vi "Top - 1.vi"(0 "OPC UA client refnum out":T1, 9 "stop":bool, 11 "error IO":errorcluster) -> (3 "Az":T2, 4 "Alt":T3, 6 "HSB":T4, 8 "Fork Panel":T5, 10 "UPS":T7, 15 "Alarm Warning":T8)   [LabVIEW 2019]
uses:
  subVIs/Alarm-Ctrl.ctl
  subVIs/UPS-Ctrl.ctl
  <vilib>/OPCUA/controls/NodeId.ctl
  subVIs/Fork Panel-Ctrl.ctl
  subVIs/HSB-Ctrl.ctl
  subVIs/Alt-Ctrl.ctl
  subVIs/Az-Ctrl.ctl
  <vilib>/OPCUA/controls/OPC UA Client Refnum.ctl
  <vilib>/OPCUA/controls/Write Variant Request.ctl
  <vilib>/OPCUA/controls/Write Status.ctl
  <vilib>/OPCUA/client/Multiple Write Variant.vi
  <vilib>/OPCUA/NI OPC UA Client.lvlib
panel:
  in  "Device.Node.Set Point":i32=1000
  out "node RU":T6[](array[typedef])
  out "node RU 2":T6[](array[typedef])
  out "node RU 3":string[](array[string])
  # "Alarm Warning"
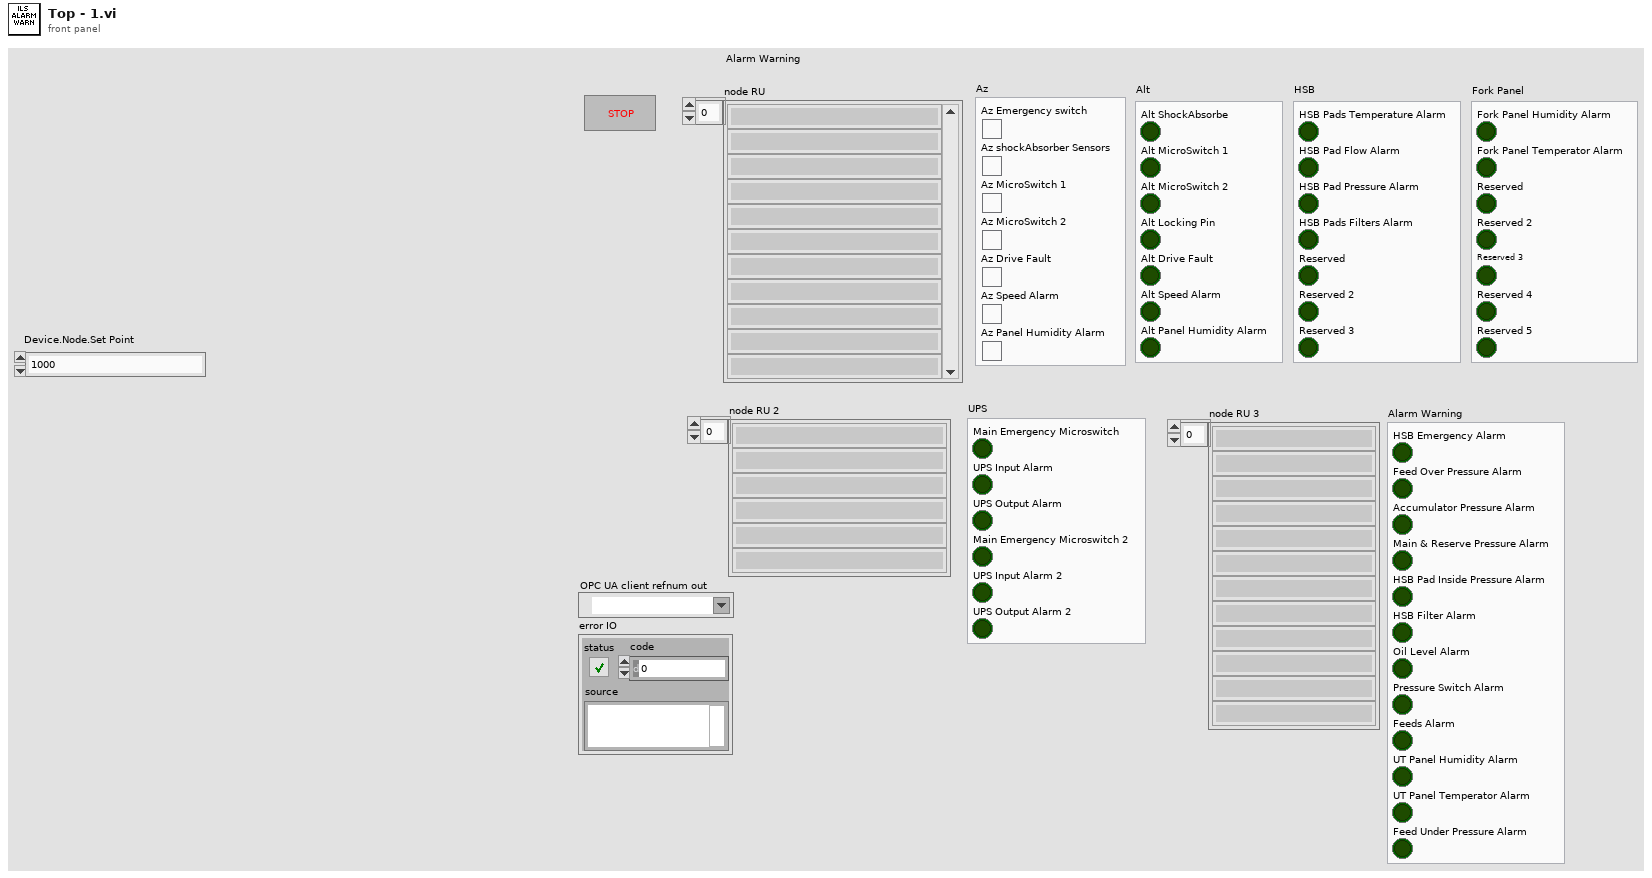
[diagram p1: front panel]
types:
  T1 = typedef "OPC UA Client Refnum.ctl" = refnum<k21>
  T2 = typedef "Az-Ctrl.ctl" = cluster{"Az Emergency switch":bool, "Az shockAbsorber Sensors":bool, "Az MicroSwitch 1":bool, "Az MicroSwitch 2":bool, "Az Drive Fault":bool, "Az Speed Alarm":bool, "Az Panel Humidity Alarm":bool}
  T3 = typedef "Alt-Ctrl.ctl" = cluster{"Alt ShockAbsorbe":bool, "Alt MicroSwitch 1":bool, "Alt MicroSwitch 2":bool, "Alt Locking Pin":bool, "Alt Drive Fault":bool, "Alt Speed Alarm":bool, "Alt Panel Humidity Alarm":bool}
  T4 = typedef "HSB-Ctrl.ctl" = cluster{"HSB Pads Temperature Alarm":bool, "HSB Pad Flow Alarm":bool, "HSB Pad Pressure Alarm":bool, "HSB Pads Filters Alarm":bool, "Reserved":bool, "Reserved 2":bool, "Reserved 3":bool}
  T5 = typedef "Fork Panel-Ctrl.ctl" = cluster{"Fork Panel Humidity Alarm":bool, "Fork Panel Temperator Alarm":bool, "Reserved":bool, "Reserved 2":bool, "Reserved 3":bool, "Reserved 4":bool, "Reserved 5":bool}
  T6 = typedef "NodeId.ctl" = string
  T7 = typedef "UPS-Ctrl.ctl" = cluster{"Main Emergency Microswitch":bool, "UPS Input Alarm":bool, "UPS Output Alarm":bool, "Main Emergency Microswitch 2":bool, "UPS Input Alarm 2":bool, "UPS Output Alarm 2":bool}
  T8 = typedef "Alarm-Ctrl.ctl" = cluster{"HSB Emergency Alarm":bool, "Feed Over Pressure Alarm":bool, "Accumulator Pressure Alarm":bool, "Main & Reserve Pressure Alarm":bool, "HSB Pad Inside Pressure Alarm":bool, "HSB Filter Alarm":bool, "Oil Level Alarm":bool, "Pressure Switch Alarm":bool, "Feeds Alarm":bool, "UT Panel Humidity Alarm":bool, "UT Panel Temperator Alarm":bool, "Feed Under Pressure Alarm":bool}
  T9 = typedef "Write Variant Request.ctl" = cluster{"node ID":T6, "value":variant, "timestamp (current time)":timestamp, "node status":T10}
  T10 = typedef "Write Status.ctl" = u32
  T11 = typedef "Subscription ID.ctl" = u32
  T12 = typedef "Subscription Data Change.ctl" = cluster{"node ID":T6, " value":variant, "timestamp":timestamp, "data type":T13, "status code":T14}
  T13 = typedef "Data Type.ctl" = u16
  T14 = typedef "OPC UA StatusCode.ctl" = u32
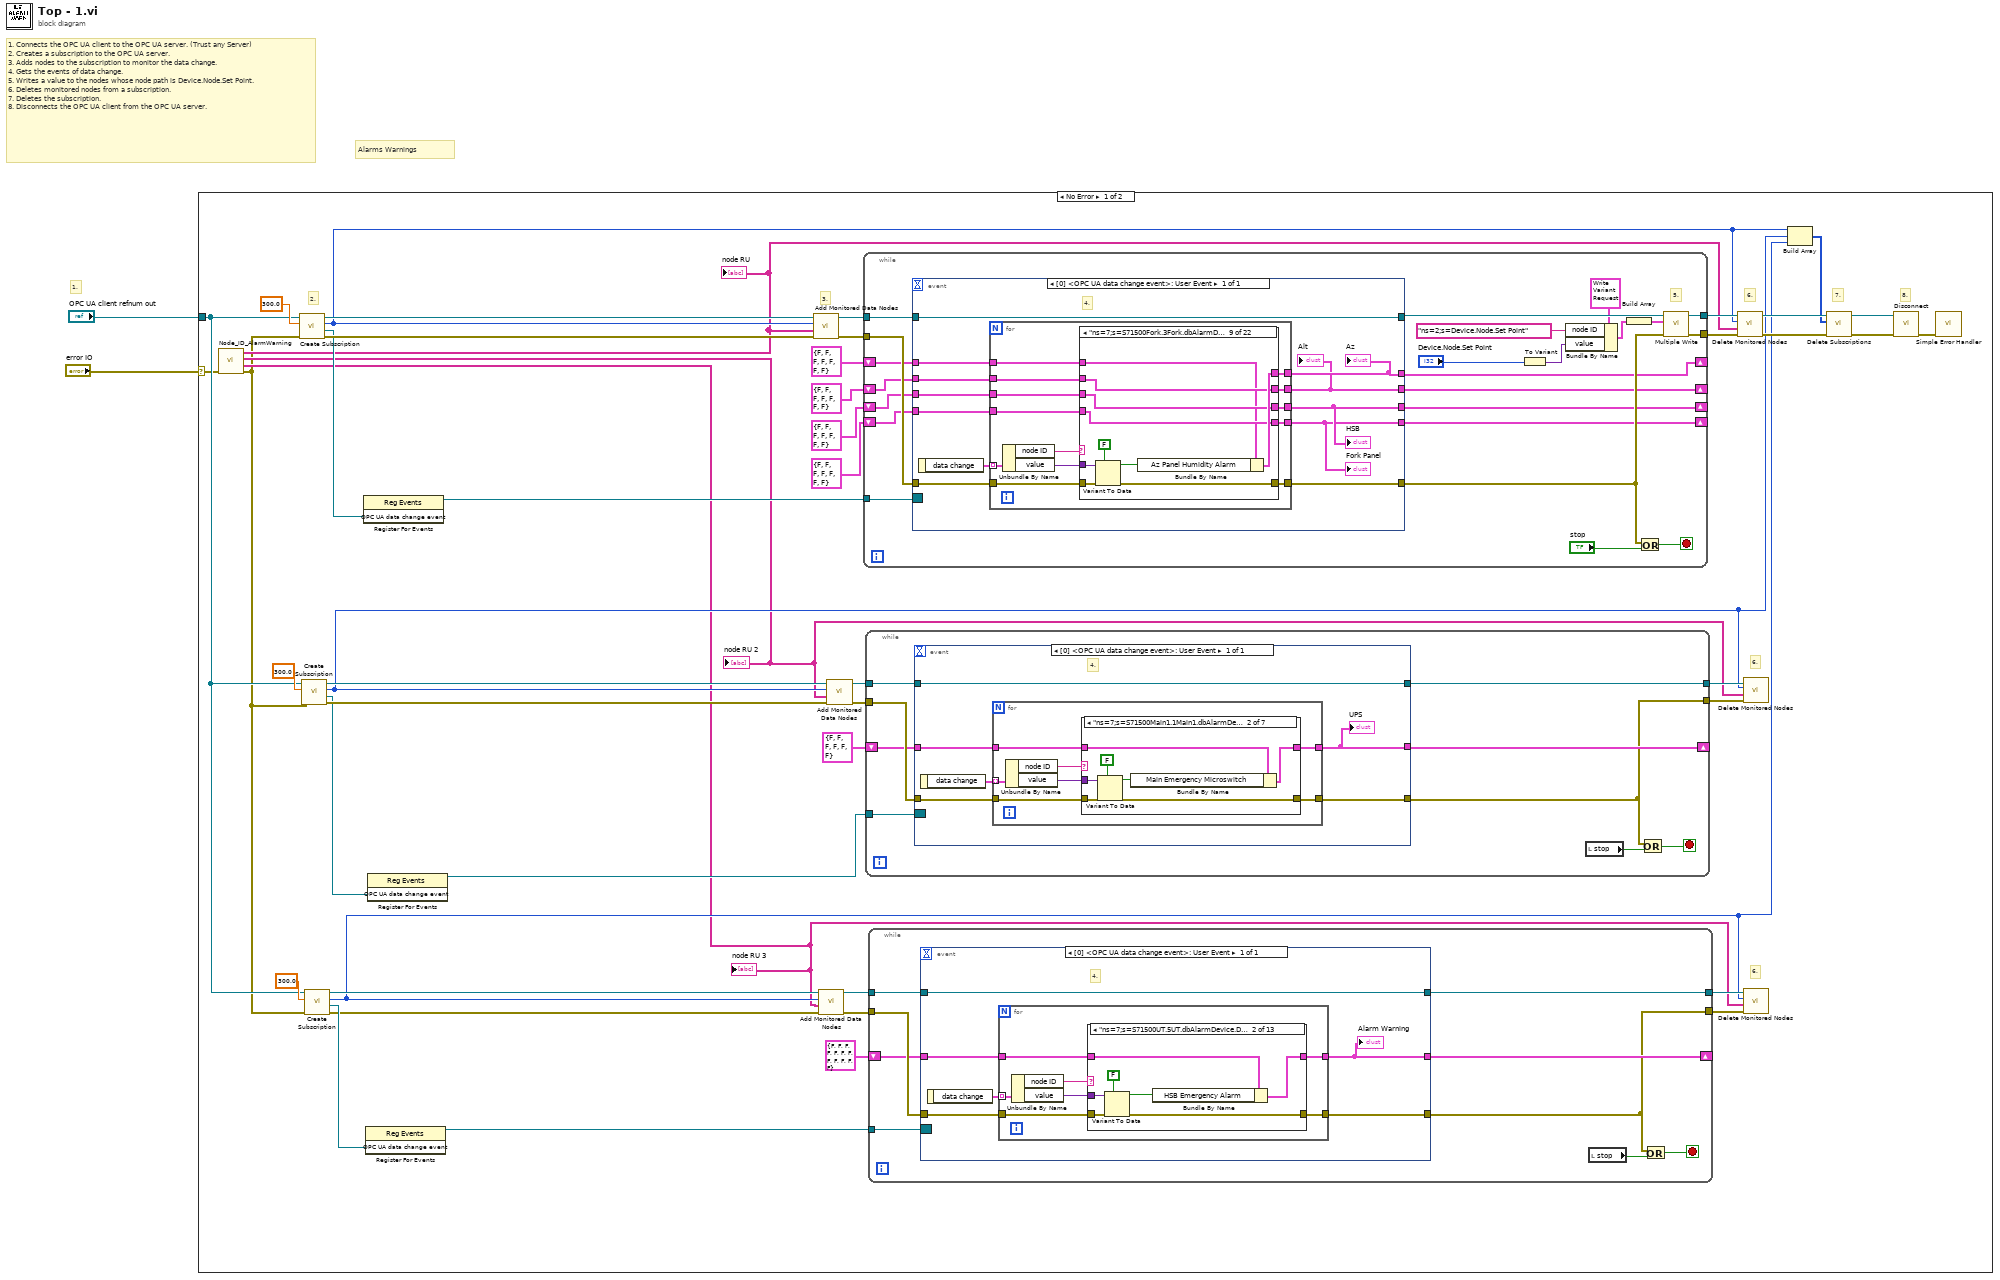
[diagram p0: block diagram]
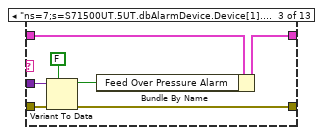
[diagram p3: hidden frame]
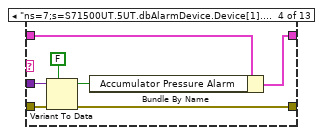
[diagram p4: hidden frame]
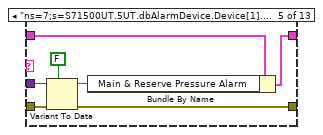
[diagram p5: hidden frame]
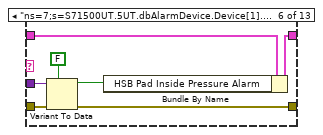
[diagram p6: hidden frame]
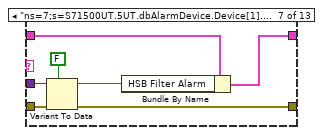
[diagram p7: hidden frame]
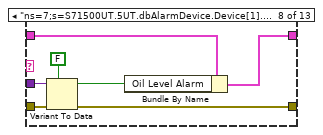
[diagram p8: hidden frame]
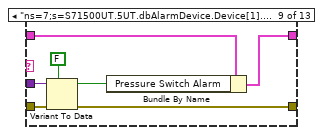
[diagram p9: hidden frame]
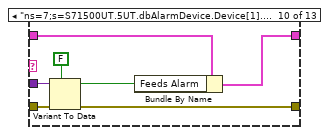
[diagram p10: hidden frame]
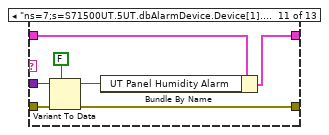
[diagram p11: hidden frame]
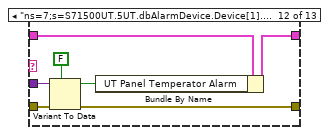
[diagram p12: hidden frame]
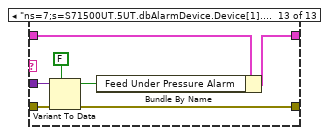
[diagram p13: hidden frame]
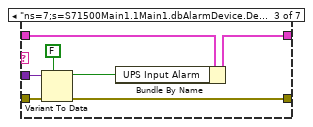
[diagram p15: hidden frame]
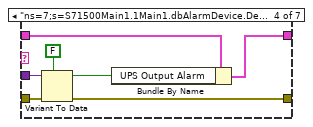
[diagram p16: hidden frame]
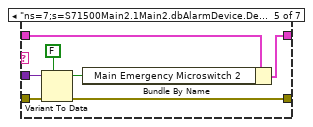
[diagram p17: hidden frame]
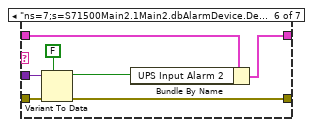
[diagram p18: hidden frame]
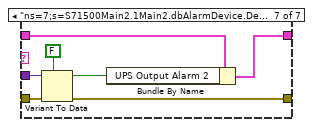
[diagram p19: hidden frame]
diagram:
  # "1."
  # "Alarms Warnings"
  # "1. Connects the OPC UA client to the OPC UA server. (Trust any Server) \n2. Creates a subscription to the OPC UA server.\n3. Adds nodes to the subscription to monitor the data change.\n4. Gets the events of data change.\n5. Writes a value to the nodes whose node path is Device.Node.Set Point. \n6. Deletes monitored nodes from a subscription.\n7. Deletes the subscription.\n8. Disconnects the OPC UA client from the OPC UA server."
  n1 = case shown="No Error" "error IO" {
    selector: "error IO" -> [w4 w487]
    tunnel: "OPC UA client refnum out" -> [w20 _]
    frame No Error {
      # "6."
      # "6."
      # "7."
      # "8."
      # "6."
      # "3."
      # "2."
      n2 = call "Node_ID_AlarmWarning.vi"("error in"=w4) -> ("error out"=w3:errorcluster, "node RU 3"=w5:string[], "node RU 2"=w6:T6[], "node RU"=w7:T6[])  [unwired: 7 in]
      "node RU" <- w7
      "node RU 2" <- w6
      "node RU 3" <- w5
      n3 = call <vilib>:"Create Subscription.vi"("error in (no error)"=w3, "publishing interval (1000 ms)"=300.0 ("update rate (1000 ms)"), "OPC UA client refnum in"=w20) -> ("error out"=w49:errorcluster, "OPC UA data change event"=w36:refnum<user-event>, "subscription ID out"=w38:T11, "OPC UA client refnum out"=w50:T1)  [unwired: 4 in, 1 out]
      n4 = call <vilib>:"Create Subscription.vi"("error in (no error)"=w3, "publishing interval (1000 ms)"=300.0, "OPC UA client refnum in"=w20) -> ("error out"=w28:errorcluster, "OPC UA data change event"=w26:refnum<user-event>, "subscription ID out"=w22:T11, "OPC UA client refnum out"=w29:T1)  [unwired: 4 in, 1 out]
      n5 = call <vilib>:"Create Subscription.vi"("error in (no error)"=w3, "publishing interval (1000 ms)"=300.0, "OPC UA client refnum in"=w20) -> ("error out"=w17:errorcluster, "OPC UA data change event"=w19:refnum<user-event>, "subscription ID out"=w11:T11, "OPC UA client refnum out"=w18:T1)  [unwired: 4 in, 1 out]
      n6 = register-events(w36) -> (reference out=w48:refnum<event-registration>)  [unwired: 2 in, 1 out]
      n7 = register-events(w19) -> (reference out=w14:refnum<event-registration>)  [unwired: 2 in, 1 out]
      n8 = register-events(w26) -> (reference out=w25:refnum<event-registration>)  [unwired: 2 in, 1 out]
      n9 = call <vilib>:"Add Monitored Data Nodes.vi"("error in (no error)"=w49, "node IDs"=w7, "subscription ID in"=w38, "OPC UA client refnum in"=w50) -> ("error out"=w46:errorcluster, "OPC UA client refnum out"=w47:T1)  [unwired: 4 in, 2 out]
      n10 = call <vilib>:"Add Monitored Data Nodes.vi"("error in (no error)"=w17, "node IDs"=w5, "subscription ID in"=w11, "OPC UA client refnum in"=w18) -> ("error out"=w15:errorcluster, "OPC UA client refnum out"=w16:T1)  [unwired: 4 in, 2 out]
      n11 = call <vilib>:"Add Monitored Data Nodes.vi"("error in (no error)"=w28, "node IDs"=w6, "subscription ID in"=w22, "OPC UA client refnum in"=w29) -> ("error out"=w27:errorcluster, "OPC UA client refnum out"=w10:T1)  [unwired: 4 in, 2 out]
      n12 = while {
        tunnel: w48 -> [w247]
        tunnel: w47 -> [w246]
        tunnel: w46 -> [w242]
        tunnel: [w243] -> w44
        tunnel: [w244] -> w45
        shift-right: [w231] -> _
        shift-left: T2 {"Az Emergency switch"=FALSE, "Az shockAbsorber Sensors"=FALSE, "Az MicroSwitch 1"=FALSE, "Az MicroSwitch 2"=FALSE, "Az Drive Fault"=FALSE, "Az Speed Alarm"=FALSE, "Az Panel Humidity Alarm"=FALSE} ("Az") -> [w232]
        shift-right: [w229] -> _
        shift-left: T3 {"Alt ShockAbsorbe"=FALSE, "Alt MicroSwitch 1"=FALSE, "Alt MicroSwitch 2"=FALSE, "Alt Locking Pin"=FALSE, "Alt Drive Fault"=FALSE, "Alt Speed Alarm"=FALSE, "Alt Panel Humidity Alarm"=FALSE} ("Cluster") -> [w230]
        shift-right: [w226] -> _
        shift-left: T4 {"HSB Pads Temperature Alarm"=FALSE, "HSB Pad Flow Alarm"=FALSE, "HSB Pad Pressure Alarm"=FALSE, "HSB Pads Filters Alarm"=FALSE, "Reserved"=FALSE, "Reserved 2"=FALSE, "Reserved 3"=FALSE} ("HSB") -> [w228]
        shift-right: [w225] -> _
        shift-left: T5 {"Fork Panel Humidity Alarm"=FALSE, "Fork Panel Temperator Alarm"=FALSE, "Reserved"=FALSE, "Reserved 2"=FALSE, "Reserved 3"=FALSE, "Reserved 4"=FALSE, "Reserved 5"=FALSE} ("Fork Panel") -> [w227]
        stop <- w235 stop-if-true
        # "5."
        n13 = event shown="[0] <OPC UA data change event>: User Event" {
          selector: w247 -> [_]
          dyn-events: _ -> [_]
          timeout: _ -> [_]
          tunnel: w246 -> [w256]
          tunnel: [w256] -> w245
          tunnel: [w257] -> w234
          tunnel: w242 -> [w258]
          tunnel: w232 -> [w255]
          tunnel: [w254] -> w231
          tunnel: w230 -> [w253]
          tunnel: [w252] -> w229
          tunnel: w228 -> [w251]
          tunnel: w227 -> [w250]
          tunnel: [w249] -> w226
          tunnel: [w248] -> w225
          event User Event {
            # "4."
            n14 = event-data() -> ("data change"=w259:T12[])  [unwired: 1 in]
            n15 = for {
              tunnel: w259 -> [w269] mode=indexing
              tunnel: w258 -> [w271]
              tunnel: [w270] -> w257
              tunnel: w255 -> [w267]
              tunnel: [w266] -> w254
              tunnel: w253 -> [w265]
              tunnel: [w264] -> w252
              tunnel: w251 -> [w263]
              tunnel: w250 -> [w261]
              tunnel: [w262] -> w249
              tunnel: [w260] -> w248
              n16 = Unbundle By Name(w269) -> ("node ID"=w268:T6, "value"=w272:variant)
              n17 = case shown="\"ns=7;s=S71500Fork.3Fork.dbAlarmDevice.Device[1].bAlarmWarning8\"" w268 {
                tunnel: w272 -> [_ w287 w297 w307 w317 w325 w335 w345 w355 w365 w375 w385 w395 w405 w415 w425 w435 w445 w455 w465 w475 w485]
                tunnel: w271 -> [w277 w285 w295 w305 w315 w323 w333 w343 w353 w363 w373 w383 w393 w403 w413 w423 w433 w443 w453 w463 w473 w483]
                tunnel: [w277 w284 w294 w304 w314 w322 w332 w342 w352 w362 w372 w382 w392 w402 w412 w422 w432 w442 w452 w462 w472 w482] -> w270
                tunnel: w267 -> [w276 w283 w293 w303 w313 w321 w331 w341 w346 w359 w369 w379 w389 w399 w409 w419 w430 w440 w450 w460 w470 w480]
                tunnel: [w276 w282 w292 w302 w312 w321 w330 w340 w351 w359 w369 w379 w389 w399 w409 w419 w430 w440 w450 w460 w470 w480] -> w266
                tunnel: w265 -> [w275 w280 w290 w300 w310 w320 w328 w338 w349 w360 w370 w380 w390 w400 w410 w420 w429 w439 w449 w459 w469 w479]
                tunnel: [w275 w280 w290 w300 w310 w320 w328 w338 w349 w358 w368 w378 w388 w398 w408 w418 w429 w439 w449 w459 w469 w479] -> w264
                tunnel: w263 -> [w274 w279 w289 w299 w309 w319 w327 w337 w348 w357 w367 w377 w387 w397 w407 w417 w428 w438 w448 w458 w468 w478]
                tunnel: [w274 w279 w289 w299 w309 w319 w327 w337 w348 w357 w367 w377 w387 w397 w407 w417 w427 w437 w447 w457 w468 w478] -> w262
                tunnel: w261 -> [w273 w278 w288 w298 w308 w318 w326 w336 w347 w356 w366 w376 w386 w396 w406 w416 w426 w436 w446 w456 w467 w477]
                tunnel: [w273 w278 w288 w298 w308 w318 w326 w336 w347 w356 w366 w376 w386 w396 w406 w416 w426 w436 w446 w456 w466 w476] -> w260
                frame "False", Default {
                }
                frame "ns=7;s=S71500Fork.3Fork.dbAlarmDevice.Device[1].bAlarmWarning1" {
                  n18 = Variant To Data(error in=w285, type=FALSE, Variant=w287) -> (data=w281:bool, error out=w284:errorcluster)
                  n19 = Bundle By Name(cluster=w283, "Az Emergency switch"=w281) -> (w282:T2)
                }
                frame "ns=7;s=S71500Fork.3Fork.dbAlarmDevice.Device[1].bAlarmWarning2" {
                  n20 = Variant To Data(error in=w295, type=FALSE, Variant=w297) -> (data=w291:bool, error out=w294:errorcluster)
                  n21 = Bundle By Name(cluster=w293, "Az shockAbsorber Sensors"=w291) -> (w292:T2)
                }
                frame "ns=7;s=S71500Fork.3Fork.dbAlarmDevice.Device[1].bAlarmWarning3" {
                  n22 = Variant To Data(error in=w305, type=FALSE, Variant=w307) -> (data=w301:bool, error out=w304:errorcluster)
                  n23 = Bundle By Name(cluster=w303, "Az MicroSwitch 1"=w301) -> (w302:T2)
                }
                frame "ns=7;s=S71500Fork.3Fork.dbAlarmDevice.Device[1].bAlarmWarning4" {
                  n24 = Variant To Data(error in=w315, type=FALSE, Variant=w317) -> (data=w311:bool, error out=w314:errorcluster)
                  n25 = Bundle By Name(cluster=w313, "Az MicroSwitch 2"=w311) -> (w312:T2)
                }
                frame "ns=7;s=S71500Fork.3Fork.dbAlarmDevice.Device[1].bAlarmWarning5" {
                  n26 = Variant To Data(error in=w323, type=FALSE, Variant=w325) -> (error out=w322:errorcluster)  [unwired: 1 out]
                }
                frame "ns=7;s=S71500Fork.3Fork.dbAlarmDevice.Device[1].bAlarmWarning6" {
                  n27 = Variant To Data(error in=w333, type=FALSE, Variant=w335) -> (data=w329:bool, error out=w332:errorcluster)
                  n28 = Bundle By Name(cluster=w331, "Az Drive Fault"=w329) -> (w330:T2)
                }
                frame "ns=7;s=S71500Fork.3Fork.dbAlarmDevice.Device[1].bAlarmWarning7" {
                  n29 = Variant To Data(error in=w343, type=FALSE, Variant=w345) -> (data=w339:bool, error out=w342:errorcluster)
                  n30 = Bundle By Name(cluster=w341, "Az Speed Alarm"=w339) -> (w340:T2)
                }
                frame "ns=7;s=S71500Fork.3Fork.dbAlarmDevice.Device[1].bAlarmWarning8" {
                  n31 = Variant To Data(error in=w353, type=FALSE, Variant=w355) -> (data=w350:bool, error out=w352:errorcluster)
                  n32 = Bundle By Name(cluster=w346, "Az Panel Humidity Alarm"=w350) -> (w351:T2)
                }
                frame "ns=7;s=S71500Fork.3Fork.dbAlarmDevice.Device[2].bAlarmWarning2" {
                  n33 = Variant To Data(error in=w363, type=FALSE, Variant=w365) -> (data=w361:bool, error out=w362:errorcluster)
                  n34 = Bundle By Name(cluster=w360, "Alt ShockAbsorbe"=w361) -> (w358:T3)
                }
                frame "ns=7;s=S71500Fork.3Fork.dbAlarmDevice.Device[2].bAlarmWarning3" {
                  n35 = Variant To Data(error in=w373, type=FALSE, Variant=w375) -> (data=w371:bool, error out=w372:errorcluster)
                  n36 = Bundle By Name(cluster=w370, "Alt MicroSwitch 1"=w371) -> (w368:T3)
                }
                frame "ns=7;s=S71500Fork.3Fork.dbAlarmDevice.Device[2].bAlarmWarning4" {
                  n37 = Variant To Data(error in=w383, type=FALSE, Variant=w385) -> (data=w381:bool, error out=w382:errorcluster)
                  n38 = Bundle By Name(cluster=w380, "Alt MicroSwitch 2"=w381) -> (w378:T3)
                }
                frame "ns=7;s=S71500Fork.3Fork.dbAlarmDevice.Device[2].bAlarmWarning5" {
                  n39 = Variant To Data(error in=w393, type=FALSE, Variant=w395) -> (data=w391:bool, error out=w392:errorcluster)
                  n40 = Bundle By Name(cluster=w390, "Alt Locking Pin"=w391) -> (w388:T3)
                }
                frame "ns=7;s=S71500Fork.3Fork.dbAlarmDevice.Device[2].bAlarmWarning6" {
                  n41 = Variant To Data(error in=w403, type=FALSE, Variant=w405) -> (data=w401:bool, error out=w402:errorcluster)
                  n42 = Bundle By Name(cluster=w400, "Alt Drive Fault"=w401) -> (w398:T3)
                }
                frame "ns=7;s=S71500Fork.3Fork.dbAlarmDevice.Device[2].bAlarmWarning7" {
                  n43 = Variant To Data(error in=w413, type=FALSE, Variant=w415) -> (data=w411:bool, error out=w412:errorcluster)
                  n44 = Bundle By Name(cluster=w410, "Alt Speed Alarm"=w411) -> (w408:T3)
                }
                frame "ns=7;s=S71500Fork.3Fork.dbAlarmDevice.Device[2].bAlarmWarning8" {
                  n45 = Variant To Data(error in=w423, type=FALSE, Variant=w425) -> (data=w421:bool, error out=w422:errorcluster)
                  n46 = Bundle By Name(cluster=w420, "Alt Panel Humidity Alarm"=w421) -> (w418:T3)
                }
                frame "ns=7;s=S71500Fork.3Fork.dbAlarmDevice.Device[3].bAlarmWarning2" {
                  n47 = Variant To Data(error in=w433, type=FALSE, Variant=w435) -> (data=w431:bool, error out=w432:errorcluster)
                  n48 = Bundle By Name(cluster=w428, "HSB Pads Temperature Alarm"=w431) -> (w427:T4)
                }
                frame "ns=7;s=S71500Fork.3Fork.dbAlarmDevice.Device[3].bAlarmWarning3" {
                  n49 = Variant To Data(error in=w443, type=FALSE, Variant=w445) -> (data=w441:bool, error out=w442:errorcluster)
                  n50 = Bundle By Name(cluster=w438, "HSB Pad Flow Alarm"=w441) -> (w437:T4)
                }
                frame "ns=7;s=S71500Fork.3Fork.dbAlarmDevice.Device[3].bAlarmWarning4" {
                  n51 = Variant To Data(error in=w453, type=FALSE, Variant=w455) -> (data=w451:bool, error out=w452:errorcluster)
                  n52 = Bundle By Name(cluster=w448, "HSB Pad Pressure Alarm"=w451) -> (w447:T4)
                }
                frame "ns=7;s=S71500Fork.3Fork.dbAlarmDevice.Device[3].bAlarmWarning5" {
                  n53 = Variant To Data(error in=w463, type=FALSE, Variant=w465) -> (data=w461:bool, error out=w462:errorcluster)
                  n54 = Bundle By Name(cluster=w458, "HSB Pads Filters Alarm"=w461) -> (w457:T4)
                }
                frame "ns=7;s=S71500Fork.3Fork.dbAlarmDevice.Device[4].bAlarmWarning8" {
                  n55 = Variant To Data(error in=w473, type=FALSE, Variant=w475) -> (data=w471:bool, error out=w472:errorcluster)
                  n56 = Bundle By Name(cluster=w467, "Fork Panel Humidity Alarm"=w471) -> (w466:T5)
                }
                frame "ns=7;s=S71500Fork.3Fork.dbAlarmDevice.Device[4].bAlarmWarning9" {
                  n57 = Variant To Data(error in=w483, type=FALSE, Variant=w485) -> (data=w481:bool, error out=w482:errorcluster)
                  n58 = Bundle By Name(cluster=w477, "Fork Panel Temperator Alarm"=w481) -> (w476:T5)
                }
              }
            }
            "Az" <- w254
            "Alt" <- w252
            "HSB" <- w249
            "Fork Panel" <- w248
          }
        }
        n59 = To Variant(anything="Device.Node.Set Point") -> (Variant=w240:variant)
        n60 = Bundle By Name(cluster=T9 {"node ID"="", "value"=variant, "timestamp (current time)"=timestamp(0 s since 1904-01-01), "node status"=0} ("request"), "node ID"=T6 "ns=2;s=Device.Node.Set Point", "value"=w240) -> (w237:T9)
        n61 = Build Array(w237) -> (w236:T9[])
        n62 = Or(x=w234, y="stop") -> (x .or. y?=w235:bool)
        n63 = call-poly <vilib>:"Multiple Write.vi"("error in (no error)"=w234, "requests"=w236, "OPC UA client refnum in"=w245) -> ("error out"=w243:errorcluster, "OPC UA client refnum out"=w244:T1)  [unwired: 5 in, 2 out]
      }
      n64 = while {
        tunnel: w25 -> [w167]
        tunnel: w10 -> [w166]
        tunnel: w27 -> [w165]
        shift-right: [w162] -> _
        shift-left: T7 {"Main Emergency Microswitch"=FALSE, "UPS Input Alarm"=FALSE, "UPS Output Alarm"=FALSE, "Main Emergency Microswitch 2"=FALSE, "UPS Input Alarm 2"=FALSE, "UPS Output Alarm 2"=FALSE} ("UPS") -> [w163]
        tunnel: [w161] -> w24
        tunnel: [w160] -> w23
        stop <- w164 stop-if-true
        n65 = event shown="[0] <OPC UA data change event>: User Event" {
          selector: w167 -> [_]
          dyn-events: _ -> [_]
          timeout: _ -> [_]
          tunnel: w166 -> [w170]
          tunnel: [w170] -> w161
          tunnel: [w171] -> w160
          tunnel: w165 -> [w172]
          tunnel: w163 -> [w169]
          tunnel: [w168] -> w162
          event User Event {
            # "4."
            n66 = event-data() -> ("data change"=w173:T12[])  [unwired: 1 in]
            n67 = for {
              tunnel: w173 -> [w177] mode=indexing
              tunnel: w172 -> [w179]
              tunnel: [w178] -> w171
              tunnel: w169 -> [w175]
              tunnel: [w174] -> w168
              n68 = Unbundle By Name(w177) -> ("node ID"=w176:T6, "value"=w180:variant)
              n69 = case shown="\"ns=7;s=S71500Main1.1Main1.dbAlarmDevice.Device[1].bAlarmWarning1\"" w176 {
                tunnel: w180 -> [_ w189 w196 w203 w210 w217 w224]
                tunnel: w179 -> [w182 w187 w194 w201 w208 w215 w222]
                tunnel: [w182 w186 w193 w200 w207 w214 w221] -> w178
                tunnel: w175 -> [w181 w185 w192 w199 w206 w212 w220]
                tunnel: [w181 w183 w191 w198 w205 w211 w219] -> w174
                frame "False", Default {
                }
                frame "ns=7;s=S71500Main1.1Main1.dbAlarmDevice.Device[1].bAlarmWarning1" {
                  n70 = Variant To Data(error in=w187, type=FALSE, Variant=w189) -> (data=w184:bool, error out=w186:errorcluster)
                  n71 = Bundle By Name(cluster=w185, "Main Emergency Microswitch"=w184) -> (w183:T7)
                }
                frame "ns=7;s=S71500Main1.1Main1.dbAlarmDevice.Device[1].bAlarmWarning2" {
                  n72 = Variant To Data(error in=w194, type=FALSE, Variant=w196) -> (data=w190:bool, error out=w193:errorcluster)
                  n73 = Bundle By Name(cluster=w192, "UPS Input Alarm"=w190) -> (w191:T7)
                }
                frame "ns=7;s=S71500Main1.1Main1.dbAlarmDevice.Device[1].bAlarmWarning3" {
                  n74 = Variant To Data(error in=w201, type=FALSE, Variant=w203) -> (data=w197:bool, error out=w200:errorcluster)
                  n75 = Bundle By Name(cluster=w199, "UPS Output Alarm"=w197) -> (w198:T7)
                }
                frame "ns=7;s=S71500Main2.1Main2.dbAlarmDevice.Device[1].bAlarmWarning1" {
                  n76 = Variant To Data(error in=w208, type=FALSE, Variant=w210) -> (data=w204:bool, error out=w207:errorcluster)
                  n77 = Bundle By Name(cluster=w206, "Main Emergency Microswitch 2"=w204) -> (w205:T7)
                }
                frame "ns=7;s=S71500Main2.1Main2.dbAlarmDevice.Device[1].bAlarmWarning2" {
                  n78 = Variant To Data(error in=w215, type=FALSE, Variant=w217) -> (data=w213:bool, error out=w214:errorcluster)
                  n79 = Bundle By Name(cluster=w212, "UPS Input Alarm 2"=w213) -> (w211:T7)
                }
                frame "ns=7;s=S71500Main2.1Main2.dbAlarmDevice.Device[1].bAlarmWarning3" {
                  n80 = Variant To Data(error in=w222, type=FALSE, Variant=w224) -> (data=w218:bool, error out=w221:errorcluster)
                  n81 = Bundle By Name(cluster=w220, "UPS Output Alarm 2"=w218) -> (w219:T7)
                }
              }
            }
            "UPS" <- w168
          }
        }
        n82 = local read "stop"() -> (w159:bool)
        n83 = Or(x=w160, y=w159) -> (x .or. y?=w164:bool)
      }
      n84 = while {
        tunnel: w14 -> [w59]
        tunnel: w16 -> [w58]
        tunnel: w15 -> [w57]
        shift-right: [w54] -> _
        shift-left: T8 {"HSB Emergency Alarm"=FALSE, "Feed Over Pressure Alarm"=FALSE, "Accumulator Pressure Alarm"=FALSE, "Main & Reserve Pressure Alarm"=FALSE, "HSB Pad Inside Pressure Alarm"=FALSE, "HSB Filter Alarm"=FALSE, "Oil Level Alarm"=FALSE, "Pressure Switch Alarm"=FALSE, "Feeds Alarm"=FALSE, "UT Panel Humidity Alarm"=FALSE, "UT Panel Temperator Alarm"=FALSE, "Feed Under Pressure Alarm"=FALSE} ("Alarm") -> [w55]
        tunnel: [w53] -> w13
        tunnel: [w52] -> w12
        stop <- w56 stop-if-true
        n85 = event shown="[0] <OPC UA data change event>: User Event" {
          selector: w59 -> [_]
          dyn-events: _ -> [_]
          timeout: _ -> [_]
          tunnel: w58 -> [w62]
          tunnel: [w62] -> w53
          tunnel: [w63] -> w52
          tunnel: w57 -> [w64]
          tunnel: w55 -> [w61]
          tunnel: [w60] -> w54
          event User Event {
            # "4."
            n86 = event-data() -> ("data change"=w65:T12[])  [unwired: 1 in]
            n87 = for {
              tunnel: w65 -> [w69] mode=indexing
              tunnel: w64 -> [w71]
              tunnel: [w70] -> w63
              tunnel: w61 -> [w67]
              tunnel: [w66] -> w60
              n88 = Unbundle By Name(w69) -> ("node ID"=w68:T6, "value"=w72:variant)
              n89 = case shown="\"ns=7;s=S71500UT.5UT.dbAlarmDevice.Device[1].bAlarmWarning1\"" w68 {
                tunnel: w72 -> [_ w81 w88 w95 w102 w109 w116 w123 w130 w137 w144 w151 w158]
                tunnel: w71 -> [w74 w79 w86 w93 w100 w107 w114 w121 w128 w135 w142 w149 w156]
                tunnel: [w74 w78 w85 w92 w99 w106 w113 w120 w127 w134 w141 w148 w155] -> w70
                tunnel: w67 -> [w73 w77 w84 w91 w98 w104 w112 w119 w126 w133 w140 w147 w154]
                tunnel: [w73 w75 w83 w90 w97 w103 w111 w118 w125 w132 w139 w146 w153] -> w66
                frame "False", Default {
                }
                frame "ns=7;s=S71500UT.5UT.dbAlarmDevice.Device[1].bAlarmWarning1" {
                  n90 = Variant To Data(error in=w79, type=FALSE, Variant=w81) -> (data=w76:bool, error out=w78:errorcluster)
                  n91 = Bundle By Name(cluster=w77, "HSB Emergency Alarm"=w76) -> (w75:T8)
                }
                frame "ns=7;s=S71500UT.5UT.dbAlarmDevice.Device[1].bAlarmWarning2" {
                  n92 = Variant To Data(error in=w86, type=FALSE, Variant=w88) -> (data=w82:bool, error out=w85:errorcluster)
                  n93 = Bundle By Name(cluster=w84, "Feed Over Pressure Alarm"=w82) -> (w83:T8)
                }
                frame "ns=7;s=S71500UT.5UT.dbAlarmDevice.Device[1].bAlarmWarning3" {
                  n94 = Variant To Data(error in=w93, type=FALSE, Variant=w95) -> (data=w89:bool, error out=w92:errorcluster)
                  n95 = Bundle By Name(cluster=w91, "Accumulator Pressure Alarm"=w89) -> (w90:T8)
                }
                frame "ns=7;s=S71500UT.5UT.dbAlarmDevice.Device[1].bAlarmWarning4" {
                  n96 = Variant To Data(error in=w100, type=FALSE, Variant=w102) -> (data=w96:bool, error out=w99:errorcluster)
                  n97 = Bundle By Name(cluster=w98, "Main & Reserve Pressure Alarm"=w96) -> (w97:T8)
                }
                frame "ns=7;s=S71500UT.5UT.dbAlarmDevice.Device[1].bAlarmWarning5" {
                  n98 = Variant To Data(error in=w107, type=FALSE, Variant=w109) -> (data=w105:bool, error out=w106:errorcluster)
                  n99 = Bundle By Name(cluster=w104, "HSB Pad Inside Pressure Alarm"=w105) -> (w103:T8)
                }
                frame "ns=7;s=S71500UT.5UT.dbAlarmDevice.Device[1].bAlarmWarning6" {
                  n100 = Variant To Data(error in=w114, type=FALSE, Variant=w116) -> (data=w110:bool, error out=w113:errorcluster)
                  n101 = Bundle By Name(cluster=w112, "HSB Filter Alarm"=w110) -> (w111:T8)
                }
                frame "ns=7;s=S71500UT.5UT.dbAlarmDevice.Device[1].bAlarmWarning7" {
                  n102 = Variant To Data(error in=w121, type=FALSE, Variant=w123) -> (data=w117:bool, error out=w120:errorcluster)
                  n103 = Bundle By Name(cluster=w119, "Oil Level Alarm"=w117) -> (w118:T8)
                }
                frame "ns=7;s=S71500UT.5UT.dbAlarmDevice.Device[1].bAlarmWarning8" {
                  n104 = Variant To Data(error in=w128, type=FALSE, Variant=w130) -> (data=w124:bool, error out=w127:errorcluster)
                  n105 = Bundle By Name(cluster=w126, "Pressure Switch Alarm"=w124) -> (w125:T8)
                }
                frame "ns=7;s=S71500UT.5UT.dbAlarmDevice.Device[1].bAlarmWarning9" {
                  n106 = Variant To Data(error in=w135, type=FALSE, Variant=w137) -> (data=w131:bool, error out=w134:errorcluster)
                  n107 = Bundle By Name(cluster=w133, "Feeds Alarm"=w131) -> (w132:T8)
                }
                frame "ns=7;s=S71500UT.5UT.dbAlarmDevice.Device[1].bAlarmWarning10" {
                  n108 = Variant To Data(error in=w142, type=FALSE, Variant=w144) -> (data=w138:bool, error out=w141:errorcluster)
                  n109 = Bundle By Name(cluster=w140, "UT Panel Humidity Alarm"=w138) -> (w139:T8)
                }
                frame "ns=7;s=S71500UT.5UT.dbAlarmDevice.Device[1].bAlarmWarning11" {
                  n110 = Variant To Data(error in=w149, type=FALSE, Variant=w151) -> (data=w145:bool, error out=w148:errorcluster)
                  n111 = Bundle By Name(cluster=w147, "UT Panel Temperator Alarm"=w145) -> (w146:T8)
                }
                frame "ns=7;s=S71500UT.5UT.dbAlarmDevice.Device[1].bAlarmWarning12" {
                  n112 = Variant To Data(error in=w156, type=FALSE, Variant=w158) -> (data=w152:bool, error out=w155:errorcluster)
                  n113 = Bundle By Name(cluster=w154, "Feed Under Pressure Alarm"=w152) -> (w153:T8)
                }
              }
            }
            "Alarm Warning" <- w60
          }
        }
        n114 = local read "stop"() -> (w51:bool)
        n115 = Or(x=w52, y=w51) -> (x .or. y?=w56:bool)
      }
      n116 = call <vilib>:"Delete Monitored Nodes.vi"("error in (no error)"=w44, "node IDs"=w7, "subscription ID in"=w38, "OPC UA client refnum in"=w45) -> ("error out"=w42:errorcluster, "OPC UA client refnum out"=w43:T1)  [unwired: 3 in, 3 out]
      n117 = call <vilib>:"Delete Monitored Nodes.vi"("error in (no error)"=w23, "node IDs"=w6, "subscription ID in"=w22, "OPC UA client refnum in"=w24) -> ()  [unwired: 3 in, 5 out]
      n118 = call <vilib>:"Delete Monitored Nodes.vi"("error in (no error)"=w12, "node IDs"=w5, "subscription ID in"=w11, "OPC UA client refnum in"=w13) -> ()  [unwired: 3 in, 5 out]
      n119 = Build Array(w38, w22, w11) -> (w37:T11[])
      n120 = call <vilib>:"Delete Subscriptions.vi"("error in (no error)"=w42, "subscription IDs"=w37, "OPC UA client refnum in"=w43) -> ("error out"=w40:errorcluster, "OPC UA client refnum out"=w41:T1)  [unwired: 6 in, 1 out]
      n121 = call <vilib>:"Disconnect.vi"("error in (no error)"=w40, "OPC UA client refnum in"=w41) -> ("error out"=w32:errorcluster)  [unwired: 9 in]
      n122 = call <vilib>:"Simple Error Handler.vi"("error in (no error)"=w32) -> ()  [unwired: 4 in, 5 out]
    }
    frame Error {
      n123 = Unbundle By Name(w487) -> ("code"=w486:i32)
      n124 = case shown="-356612" w486 {
        frame 0, Default {
        }
        frame -356612 {
          n125 = One Button Dialog(message="A communication problem occurred. Ensure that the OPC UA server that you specify in the server endpoint URL is running and the network between the OPC UA server and the OPC UA client is connectable.") -> ()  [unwired: 1 in, 1 out]
        }
      }
    }
  }
